vi "CONFIG NEO LIMITS.vi"(8 "error in (no error)":errorcluster, 9 "MotorControlDeviceRef in":T1, 10 "Enable SOFT LIMIT? (T)":bool=TRUE, 11 "Enable HARD LIMIT? (T)":bool=TRUE) -> (0 "error out":errorcluster, 3 "MotorControlDeviceRef out":T1)   [LabVIEW 2020]
uses:
  <vilib>/Rock Robotics/WPI/MotorControl/WPI_MotorControlDeviceRef.ctl
  <vilib>/Rock Robotics/WPI/MotorControl/WPI_MotorControlType.ctl
  <vilib>/Rock Robotics/SystemInterfaces/DIO/FPGA_DIOPWMChannel.ctl
  <vilib>/Rock Robotics/WPI/PWM/WPI_PWMDeadband.ctl
  <vilib>/Rock Robotics/SystemInterfaces/DIO/FPGA_DIOChannel.ctl
  <vilib>/Rock Robotics/WPI/ThirdParty/REV Robotics/REVLib/Typedef/Spark MAX Limit Direction.ctl
  <vilib>/Rock Robotics/WPI/ThirdParty/REV Robotics/REVLib/Typedef/Spark MAX Limit Switch Polarity.ctl
  Robot Global Data.vi
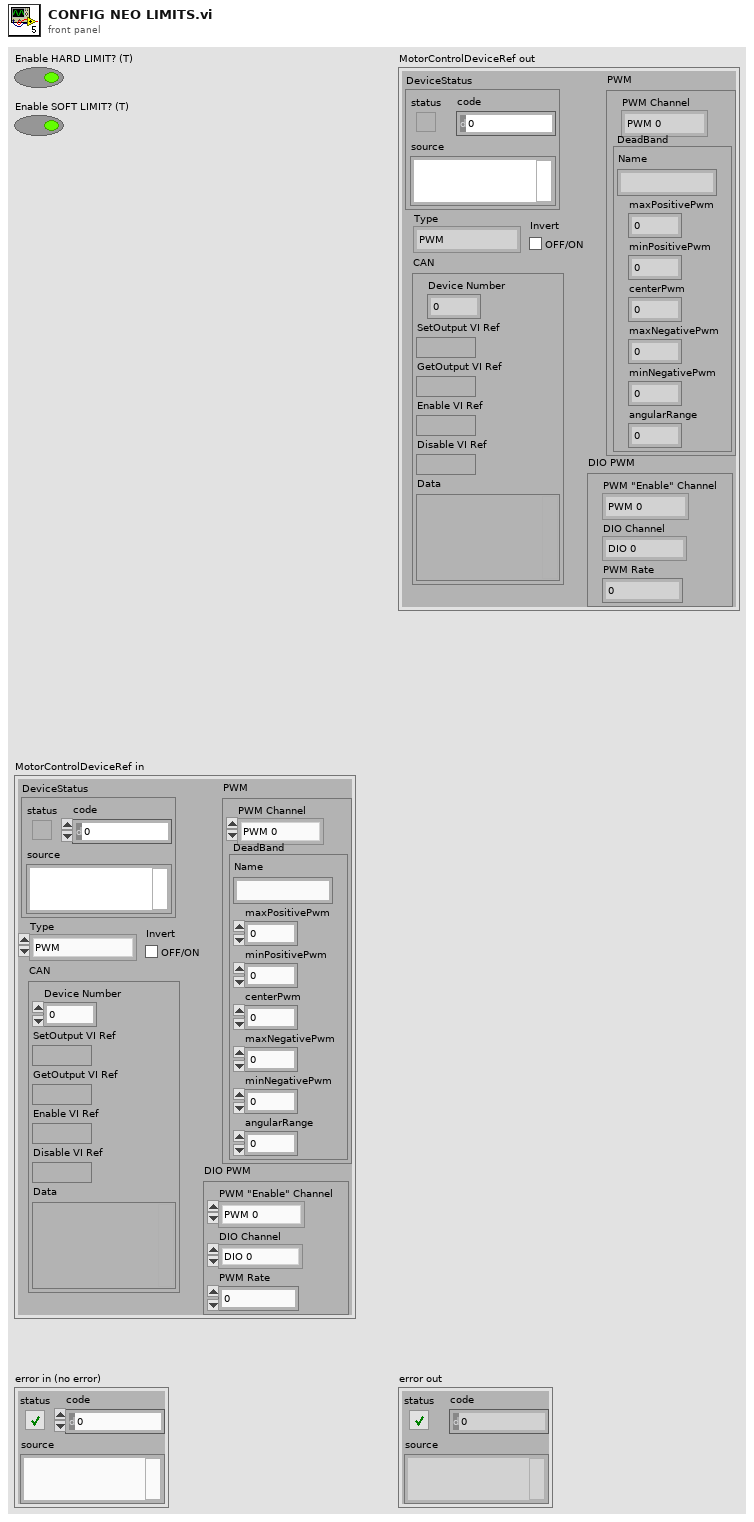
[diagram p1: front panel]
types:
  T1 = typedef "WPI_MotorControlDeviceRef.ctl" = cluster{"DeviceStatus":errorcluster, "Type":T2, "PWM":cluster{"PWM Channel":T3, "DeadBand":T4}, "CAN":cluster{"Device Number":u8, "SetOutput VI Ref":variant, "GetOutput VI Ref":variant, "Enable VI Ref":variant, "Disable VI Ref":variant, "Data":variant}, "Invert":bool, "DIO PWM":cluster{"PWM \"Enable\" Channel":T3, "DIOChannel":T5, "PWM Rate":dbl}}
  T2 = typedef "WPI_MotorControlType.ctl" = enum16{"PWM", "CAN", "DIO PWM"}
  T3 = typedef "FPGA_DIOPWMChannel.ctl" = enum8{"PWM 0", "PWM 1", "PWM 2", "PWM 3", "PWM 4", "PWM 5", "PWM 6", "PWM 7", "PWM 8", "PWM 9", "PWM MXP 0", "PWM MXP 1", "PWM MXP 2", "PWM MXP 3", "PWM MXP 4", "PWM MXP 5", "PWM MXP 6", "PWM MXP 7", "PWM MXP 8", "PWM MXP 9", "Invalid"}
  T4 = typedef "WPI_PWMDeadband.ctl" = cluster{"Name":string, "maxPositivePwm":i32, "minPositivePwm":i32, "centerPwm":i32, "maxNegativePwm":i32, "minNegativePwm":i32, "angularRange":u16}
  T5 = typedef "FPGA_DIOChannel.ctl" = enum8{"DIO 0", "DIO 1", "DIO 2", "DIO 3", "DIO 4", "DIO 5", "DIO 6", "DIO 7", "DIO 8", "DIO 9", "DIO MXP 0", "DIO MXP 1", "DIO MXP 2", "DIO MXP 3", "DIO MXP 4", "DIO MXP 5", "DIO MXP 6", "DIO MXP 7", "DIO MXP 8", "DIO MXP 9", "DIO MXP 10", "DIO MXP 11", "DIO MXP 12", "DIO MXP 13", "DIO MXP 14", "DIO MXP 15", "SPI Port CS1", "SPI Port CS2", "SPI Port CS3", "SPI Port MISO", "SPI Port MOSI", "Invalid"}
  T6 = typedef "Spark MAX Limit Switch Polarity.ctl" = enum16{"Normally Open", "Normally Closed"}
  T7 = cluster{"MIN":dbl, "MAX":dbl, "convert arm inches to revs":dbl, "convert arm inches to degrees":dbl}
  T8 = typedef "Spark MAX Limit Direction.ctl" = enum16{"Forward Limit", "Reverse Limit"}
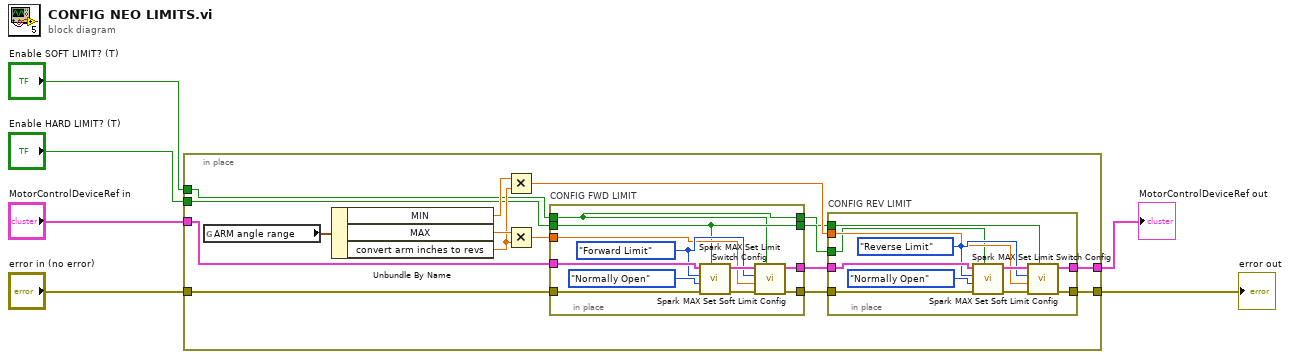
[diagram p0: block diagram]
diagram:
  n1 = in-place {
    in-place-border: [w22] -> w1
    in-place-border: "MotorControlDeviceRef in" -> [w21]
    in-place-border: "error in (no error)" -> [w20]
    in-place-border: [w17] -> w4
    in-place-border: "Enable HARD LIMIT? (T)" -> [w10]
    in-place-border: "Enable SOFT LIMIT? (T)" -> [w8]
    n2 = global read "Robot Global Data.vi" "ARM angle range"() -> (w11:T7)
    n3 = Unbundle By Name(w11) -> ("MIN"=w12:dbl, "MAX"=w15:dbl, "convert arm inches to revs"=w13:dbl)
    n4 = Multiply(x=w12, y=w13) -> (x*y=w14:dbl)
    n5 = Multiply(x=w15, y=w13) -> (x*y=w16:dbl)
    n6 = in-place "CONFIG FWD LIMIT" {
      in-place-border: w21 -> [w44]
      in-place-border: w20 -> [w43]
      in-place-border: [w41] -> w19
      in-place-border: [w39] -> w18
      in-place-border: w16 -> [w36]
      in-place-border: w10 -> [w35]
      in-place-border: [w35] -> w9
      in-place-border: w8 -> [w34]
      in-place-border: [w34] -> w7
      w37 = Spark_MAX_Limit_Direction."Forward Limit" ("Soft Limit Switch")
      n7 = call <vilib>:"Spark MAX Set Limit Switch Config.vi"("Enabled? (T)"=w35, "error in (no error)"=w43, "Polarity (Normally Open)"=Spark_MAX_Limit_Switch_Polarity."Normally Open", "Limit Switch"=w37, "MotorControlDeviceRef in"=w44) -> ("error out"=w40:errorcluster, "MotorControlDeviceRef out"=w42:T1)  [unwired: 5 in]
      n8 = call <vilib>:"Spark MAX Set Soft Limit Config.vi"("Enabled? (T)"=w34, "error in (no error)"=w40, "Soft Limit (0)"=w36, "Soft Limit Switch"=w37, "MotorControlDeviceRef in"=w42) -> ("error out"=w39:errorcluster, "MotorControlDeviceRef out"=w41:T1)  [unwired: 5 in]
    }
    n9 = in-place "CONFIG REV LIMIT" {
      in-place-border: [w29] -> w22
      in-place-border: w19 -> [w33]
      in-place-border: w18 -> [w32]
      in-place-border: [w30] -> w17
      in-place-border: w14 -> [w25]
      in-place-border: w9 -> [w24]
      in-place-border: w7 -> [w23]
      w26 = Spark_MAX_Limit_Direction."Reverse Limit" ("Soft Limit Switch")
      n10 = call <vilib>:"Spark MAX Set Limit Switch Config.vi"("Enabled? (T)"=w24, "error in (no error)"=w32, "Polarity (Normally Open)"=Spark_MAX_Limit_Switch_Polarity."Normally Open", "Limit Switch"=w26, "MotorControlDeviceRef in"=w33) -> ("error out"=w28:errorcluster, "MotorControlDeviceRef out"=w31:T1)  [unwired: 5 in]
      n11 = call <vilib>:"Spark MAX Set Soft Limit Config.vi"("Enabled? (T)"=w23, "error in (no error)"=w28, "Soft Limit (0)"=w25, "Soft Limit Switch"=w26, "MotorControlDeviceRef in"=w31) -> ("error out"=w29:errorcluster, "MotorControlDeviceRef out"=w30:T1)  [unwired: 5 in]
    }
  }
  "MotorControlDeviceRef out" <- w4
  "error out" <- w1
